vi "Xml_Write_Hardware.vi"(8 "error in (no error)":errorcluster, 11 "Variant":variant) -> (0 "error out":errorcluster, 2 "XML String Out":string[](array[string]), 3 "Variant Output":variant)   [LabVIEW 2024]
doc: "This VI reads an XML file of parameters and casts the Resource Name (String) to an IVI Class, as the GXML Lib is unable to read/write objects of type IVI class."
uses:
  <instrlib>/niHSDIO/niHSDIO.llb/niHSDIO_ctl Trigger Source Values (Ring).ctl
  <instrlib>/niScope/Controls/niScope trigger source.ctl
  <instrlib>/niFgen/niFgen.llb/niFgen_ctl Trigger Source Values (Ring).ctl
  controls/HARDWARE_Inputs.ctl
  controls/AO_6711_Inputs.ctl
  controls/AO_6738_Inputs.ctl
  controls/AWG_5421_Inputs.ctl
  controls/DIGIT_5122_Inputs.ctl
  controls/HSDIO_6541_Inputs.ctl
  <vilib>/NI/GXML/GXML.lvlib
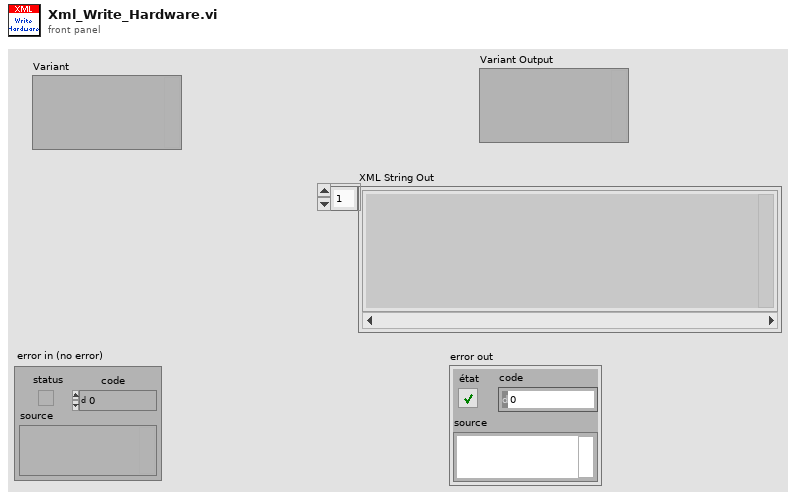
[diagram p1: front panel]
types:
  T1 = typedef "HARDWARE_Inputs.ctl" = cluster{"AO 6711 Inputs":T2, "AO 6738 Inputs":T3, "AWG 5421 Inputs":T4, "DIGIT 5122 Inputs":T6, "HSDIO 6541 Inputs":T8}
  T2 = typedef "AO_6711_Inputs.ctl" = cluster{"Physical Channels":tag, "Min Voltage":dbl, "Max Voltage":dbl, "Trigger Source":tag, "Counter":tag}
  T3 = typedef "AO_6738_Inputs.ctl" = cluster{"Physical Channels":tag, "Min Voltage":dbl, "Max Voltage":dbl, "Trigger Source":tag, "Counter":tag}
  T4 = typedef "AWG_5421_Inputs.ctl" = cluster{"Resource Name":refnum<k15>, "Sample Rate":dbl, "Trigger Type":u16, "Trigger Source":T5, "Waveform Gain":dbl, "Digital Filter ON":bool}
  T5 = typedef "niFgen_ctl Trigger Source Values (Ring).ctl" = string
  T6 = typedef "DIGIT_5122_Inputs.ctl" = cluster{"Sample Rate":dbl, "Resource Name":refnum<k15>, "Channel Name":string, "Trigger Source":T7, "Vertical Range":dbl, "Trigger Level":dbl}
  T7 = typedef "niScope trigger source.ctl" = string
  T8 = typedef "HSDIO_6541_Inputs.ctl" = cluster{"Resource Name":refnum<k15>, "Clock Rate":dbl, "Trigger Source":T9}
  T9 = typedef "niHSDIO_ctl Trigger Source Values (Ring).ctl" = string
  T10 = cluster{"Resource Name":string, "Sample Rate":dbl, "Trigger Type":u16, "Trigger Source":T5, "Waveform Gain":dbl, "Digital Filter ON":bool}
  T11 = cluster{"Sample Rate":dbl, "Resource Name":string, "Channel Name":string, "Trigger Source":T7, "Vertical Range":dbl, "Trigger Level":dbl}
  T12 = cluster{"Resource Name":string, "Clock Rate":dbl, "Trigger Source":T9}
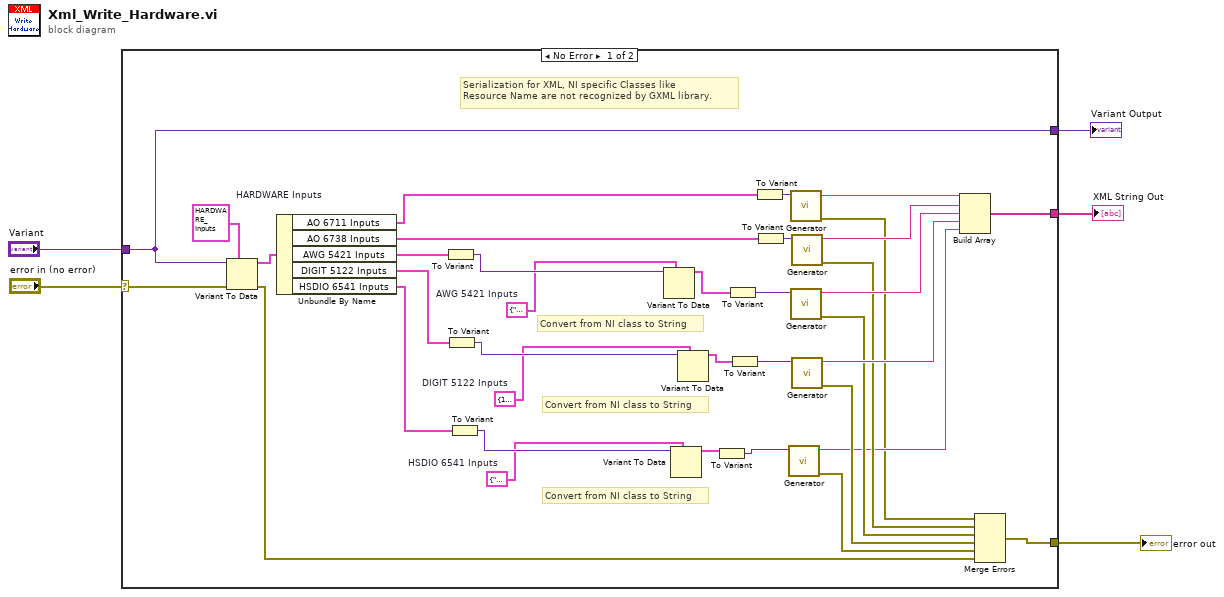
[diagram p0: block diagram]
diagram:
  n1 = case shown="No Error" "error in (no error)" {
    selector: "error in (no error)" -> [w41 w43]
    tunnel: [w40 w43] -> w4
    tunnel: [w22 w42] -> w3
    tunnel: "Variant" -> [w22 w42]
    tunnel: [w39 _] -> w1
    frame No Error {
      w38 = T1 {"AO 6711 Inputs"={"Physical Channels"="AnalogOutput/ao0:3", "Min Voltage"=-10.0, "Max Voltage"=10.0, "Trigger Source"="/AnalogOutput/PFI0", "Counter"="AnalogOutput/ctr0"}, "AO 6738 Inputs"={"Physical Channels"="AO_6738/ao0:3", "Min Voltage"=-10.0, "Max Voltage"=10.0, "Trigger Source"="/AO_6738/PFI2", "Counter"="AO_6738/ctr0"}, "AWG 5421 Inputs"={"Resource Name"="AnalogOutput/ao0:3", "Sample Rate"=20000000.0, "Trigger Type"=2, "Trigger Source"="PFI0", "Waveform Gain"=0.31, "Digital Filter ON"=TRUE}, "DIGIT 5122 Inputs"={"Sample Rate"=9.0, "Resource Name"="Digitizer", "Channel Name"="PFI0", "Trigger Source"="VAL_EXTERNAL", "Vertical Range"=10.0, "Trigger Level"=3.0}, "HSDIO 6541 Inputs"={"Resource Name"="SequencerHSDIO", "Clock Rate"=1000000.0, "Trigger Source"="PFI0"}}  # HARDWARE Inputs
      w10 = T10 {"Resource Name"="AWG_5421", "Sample Rate"=10000000.0, "Trigger Type"=2, "Trigger Source"="PFI0", "Waveform Gain"=0.31, "Digital Filter ON"=TRUE}  # AWG 5421 Inputs
      w15 = T11 {"Sample Rate"=10000.0, "Resource Name"="DIGIT_5122", "Channel Name"="0", "Trigger Source"="VAL_EXTERNAL", "Vertical Range"=10.0, "Trigger Level"=3.0}  # DIGIT 5122 Inputs
      w20 = T12 {"Resource Name"="HSDIO_6541", "Clock Rate"=1000000.0, "Trigger Source"="PFI0"}  # HSDIO 6541 Inputs
      # "Serialization for XML, NI specific Classes like\nResource Name are not recognized by GXML library."
      # "Convert from NI class to String"
      # "Convert from NI class to String"
      # "Convert from NI class to String"
      n2 = Variant To Data(error in=w41, type=w38, Variant=w22) -> (data=w37:T1, error out=w28:errorcluster)
      n3 = Unbundle By Name(w37) -> ("AO 6711 Inputs"=w8:T2, "AO 6738 Inputs"=w35:T3, "AWG 5421 Inputs"=w25:T4, "DIGIT 5122 Inputs"=w24:T6, "HSDIO 6541 Inputs"=w23:T8)
      n4 = To Variant(anything=w25) -> (Variant=w11:variant)
      n5 = To Variant(anything=w24) -> (Variant=w16:variant)
      n6 = To Variant(anything=w23) -> (Variant=w21:variant)
      n7 = Variant To Data(type=w10, Variant=w11) -> (data=w13:T10)  [unwired: 1 in, 1 out]
      n8 = Variant To Data(type=w20, Variant=w21) -> (data=w19:T12)  [unwired: 1 in, 1 out]
      n9 = Variant To Data(type=w15, Variant=w16) -> (data=w17:T11)  [unwired: 1 in, 1 out]
      n10 = To Variant(anything=w19) -> (Variant=w18:variant)
      n11 = To Variant(anything=w13) -> (Variant=w12:variant)
      n12 = To Variant(anything=w17) -> (Variant=w14:variant)
      n13 = To Variant(anything=w8) -> (Variant=w9:variant)
      n14 = To Variant(anything=w35) -> (Variant=w36:variant)
      n15 = call <vilib>:"Generator.vi"("Variant"=w18) -> ("error out"=w26:errorcluster, "XML String Out"=w27:string)  [unwired: 9 in]
      n16 = call <vilib>:"Generator.vi"("Variant"=w9) -> ("error out"=w7:errorcluster, "XML String Out"=w6:string)  [unwired: 9 in]
      n17 = call <vilib>:"Generator.vi"("Variant"=w12) -> ("error out"=w30:errorcluster, "XML String Out"=w33:string)  [unwired: 9 in]
      n18 = call <vilib>:"Generator.vi"("Variant"=w36) -> ("error out"=w31:errorcluster, "XML String Out"=w34:string)  [unwired: 9 in]
      n19 = call <vilib>:"Generator.vi"("Variant"=w14) -> ("error out"=w29:errorcluster, "XML String Out"=w32:string)  [unwired: 9 in]
      n20 = Build Array(w6, w34, w33, w32, w27) -> (w39:string[])
      n21 = Merge Errors(w7, w31, w30, w29, w26, w28) -> (w40:errorcluster)
    }
    frame Error {
    }
  }
  "error out" <- w4
  "Variant Output" <- w3
  "XML String Out" <- w1
